vi "Ultrasonic Tester.vi"() -> ()   [LabVIEW 2013]
uses:
  <vilib>/Rock Robotics/SystemInterfaces/AI/FPGA_AIChannel.ctl
panel:
  out "Numeric":i32
  in  "Left":T1=enum."AI 3"
  out "Right Distance 2":dbl
  out "Left Waveform Chart":dbl(graph)
  out "Left distance":dbl(slide)=125.0 scale=0.0..250.0 scale format="%3d"
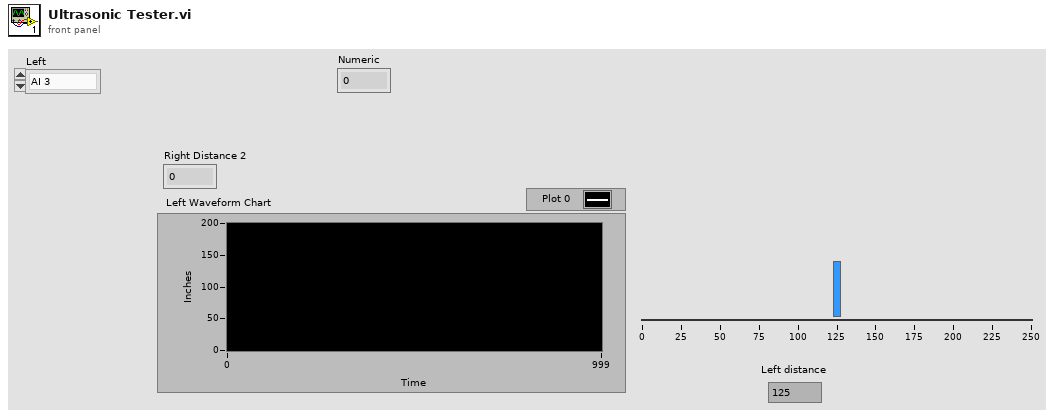
[diagram p1: front panel]
types:
  T1 = typedef "FPGA_AIChannel.ctl" = enum8{"AI 1", "AI 2", "AI 3", "AI 4", "AI 5", "AI 6", "AI 7", "AI 8", "Invalid"}
  T2 = typedef "WPI_AnalogChannelDevRef.ctl" = cluster{"DevStatus":errorcluster, "Analog Module":T3, "Analog Channel":T1}
  T3 = typedef "FPGA_TypedefAnalogModule.ctl" = enum16{"Analog Module 1", "Analog Module 2"}
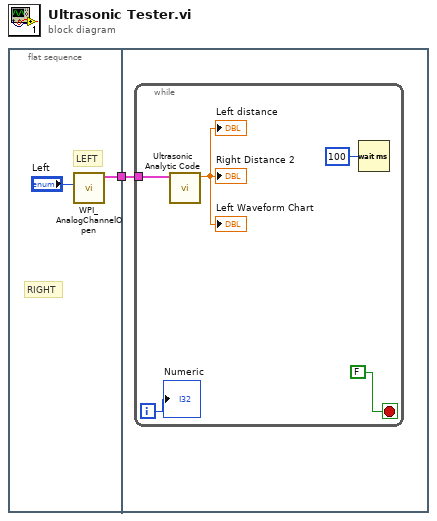
[diagram p0: block diagram]
diagram:
  n1 = flat-sequence {
    tunnel: [w2] -> w1
    tunnel: w1 -> [w4]
    frame #0 {
      # "LEFT"
      # "RIGHT"
      n2 = call <vilib>:"WPI_AnalogChannelOpen.vi"("Analog Channel"="Left") -> ("AIDeviceRef"=w2:T2)  [unwired: 2 in, 8 out]
    }
    frame #1 {
      n3 = while {
        tunnel: w4 -> [w8]
        i -> [w6]
        stop <- FALSE stop-if-true
        n4 = call "Ultrasonic Analytic Code.vi"("AIDeviceRef 2"=w8) -> ("Distance"=→"Left distance" →"Left Waveform Chart" →"Right Distance 2":dbl)  [unwired: 9 in, 1 out]
        n5 = Wait (ms)(milliseconds to wait=u32 100) -> ()  [unwired: 1 out]
        "Numeric" <- w6
      }
    }
  }
